vi "Parse Link.vi"(10 "Outputs (All)":i32, 11 "String":string) -> (3 "Routes":i32[](array[numeric]))   [LabVIEW 2022 SP3, in "VideoMux.lvlib" / "Mux.lvclass"]
uses:
  Mux.lvclass
  <vilib>/Utility/error.llb/Trim Whitespace One-Sided.vi
  <vilib>/regexp/Match Regular Expression.xnode
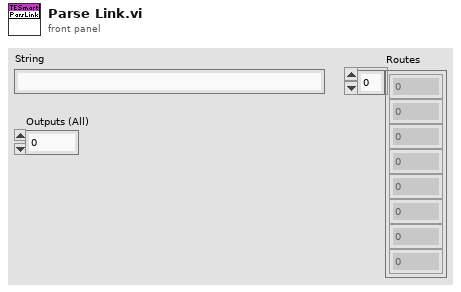
[diagram p1: front panel]
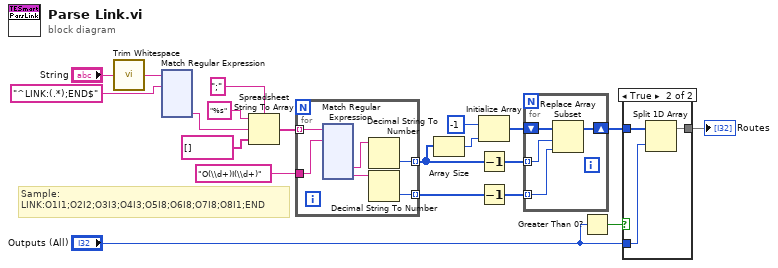
[diagram p0: block diagram]
diagram:
  # "Sample:\nLINK:O1I1;O2I2;O3I3;O4I3;O5I8;O6I8;O7I8;O8I1;END"
  n1 = call <vilib>:"Trim Whitespace.vi"("string"="String") -> ("trimmed string"=w3:string)  [unwired: 1 in]
  n2 = xnode "Match Regular Expression"("input string"=w3, "regular expression"="^LINK:(.*);END$") -> ("submatch 1"=w18:string)  [unwired: 4 in, 5 out]
  n3 = Spreadsheet String To Array(delimiter (Tab)=";", format string="%s", spreadsheet string=w18, array type (2D Dbl)=string[] []) -> (array=w14:string[])
  n4 = for {
    tunnel: w14 -> [w26] mode=indexing
    tunnel: "O(\\d+)I(\\d+)" -> [w25]
    tunnel: [w22] -> w9 mode=indexing
    tunnel: [w21] -> w8 mode=indexing
    n5 = xnode "Match Regular Expression"("input string"=w26, "regular expression"=w25) -> ("submatch 1"=w23:string, "submatch 2"=w24:string)  [unwired: 4 in, 5 out]
    n6 = Decimal String To Number(string=w23) -> (number=w22:i32)  [unwired: 2 in, 1 out]
    n7 = Decimal String To Number(string=w24) -> (number=w21:i32)  [unwired: 2 in, 1 out]
  }
  n8 = Array Size(array=w9) -> (size(s)=w12:i32)
  n9 = Initialize Array(-1 ("element"), w12) -> (w10:i32[])
  n10 = Decrement(x=w9) -> (x-1=w2:i32[])
  n11 = Decrement(x=w8) -> (x-1=w1:i32[])
  n12 = for {
    shift-right: [w147] -> w7
    shift-left: w10 -> [w150]
    tunnel: w2 -> [w149] mode=indexing
    tunnel: w1 -> [w148] mode=indexing
    n13 = Replace Array Subset(array=w150, new element=w148, index=w149) -> (w147:i32[])
  }
  n14 = Greater Than 0?(x="Outputs (All)") -> (x > 0?=w6:bool)
  n15 = case shown="True" w6 {
    tunnel: w7 -> [w151 w154]
    tunnel: "Outputs (All)" -> [_ w153]
    tunnel: [w151 w152] -> w4
    frame False {
    }
    frame True {
      n16 = Split 1D Array(array=w154, index=w153) -> (first subarray=w152:i32[])  [unwired: 1 out]
    }
  }
  "Routes" <- w4
